vi "SW_Load_settings_to_main_tab.vi"(0 "Refnum in":T3=refnum, 1 "User Name":string="Admin", 7 "error in (no error)":errorcluster) -> (9 "VISA resource name":string, 12 "Vertical offset":dbl, 13 "Midfield segments outer radius, mm":i32=60, 14 "Cage diameter, mm":i32=180, 15 "Midfield segments starting angle":i32, 16 "Border segments starting angle":i32, 17 "Stimulus presets array":T2(array[cluster])=[{"Event type"=0, "Dur., s"=0.0, "Stim., s"=0.0, "Set/Clear"=FALSE, "TTL out N"=1, "Stim. has been set"=FALSE}, {"Event type"=0, "Dur., s"=0.0, "Stim., s"=0.0, "Set/Clear"=FALSE, "TTL out N"=1, "Stim. has been set"=FALSE}, {"Event type"=0, "Dur., s"=0.0, "Stim., s"=0.0, "Set/Clear"=FALSE, "TTL out N"=1, "Stim. has been set"=FALSE}, {"Event type"=0, "Dur., s"=0.0, "Stim., s"=0.0, "Set/Clear"=FALSE, "TTL out N"=1, "Stim. has been set"=FALSE}, {"Event type"=0, "Dur., s"=0.0, "Stim., s"=0.0, "Set/Clear"=FALSE, "TTL out N"=1, "Stim. has been set"=FALSE}, {"Event type"=0, "Dur., s"=0.0, "Stim., s"=0.0, "Set/Clear"=FALSE, "TTL out N"=1, "Stim. has been set"=FALSE}, {"Event type"=0, "Dur., s"=0.0, "Stim., s"=0.0, "Set/Clear"=FALSE, "TTL out N"=1, "Stim. has been set"=FALSE}, {"Event type"=0, "Dur., s"=0.0, "Stim., s"=0.0, "Set/Clear"=FALSE, "TTL out N"=1, "Stim. has been set"=FALSE}, {"Event type"=0, "Dur., s"=0.0, "Stim., s"=0.0, "Set/Clear"=FALSE, "TTL out N"=1, "Stim. has been set"=FALSE}, {"Event type"=0, "Dur., s"=0.0, "Stim., s"=0.0, "Set/Clear"=FALSE, "TTL out N"=1, "Stim. has been set"=FALSE}, {"Event type"=0, "Dur., s"=0.0, "Stim., s"=0.0, "Set/Clear"=FALSE, "TTL out N"=1, "Stim. has been set"=FALSE}, {"Event type"=0, "Dur., s"=0.0, "Stim., s"=0.0, "Set/Clear"=FALSE, "TTL out N"=1, "Stim. has been set"=FALSE}, {"Event type"=0, "Dur., s"=0.0, "Stim., s"=0.0, "Set/Clear"=FALSE, "TTL out N"=1, "Stim. has been set"=FALSE}, {"Event type"=0, "Dur., s"=0.0, "Stim., s"=0.0, "Set/Clear"=FALSE, "TTL out N"=1, "Stim. has been set"=FALSE}] {"Event type" items=["Stay for N seconds"]; "TTL out N" items=["1"=1, "2"=2, "1+2"=3]}, 19 "IO parameters cluster":T1, 20 "Refnum out":T3, 21 "Amount of midfield segments":i32=4, 23 "Mouse snout orientation swap?":bool, 24 "Amount of border segments":i32=8, 25 "Center segment outer radius, mm":i32=30, 27 "error out":errorcluster={"status"=TRUE, "code"=1, "source"="Dequeue Element in NI_LVConfig.lvlib:Read Value Without Comment.vi->NI_LVConfig.lvlib:Read Key (I32).vi->SW_Load_settings_to_main_tab.vi"})   [LabVIEW 2016]
uses:
  <vilib>/Utility/config.llb/Config Data RefNum.ctl
  <vilib>/Utility/config.llb/NI_LVConfig.lvlib
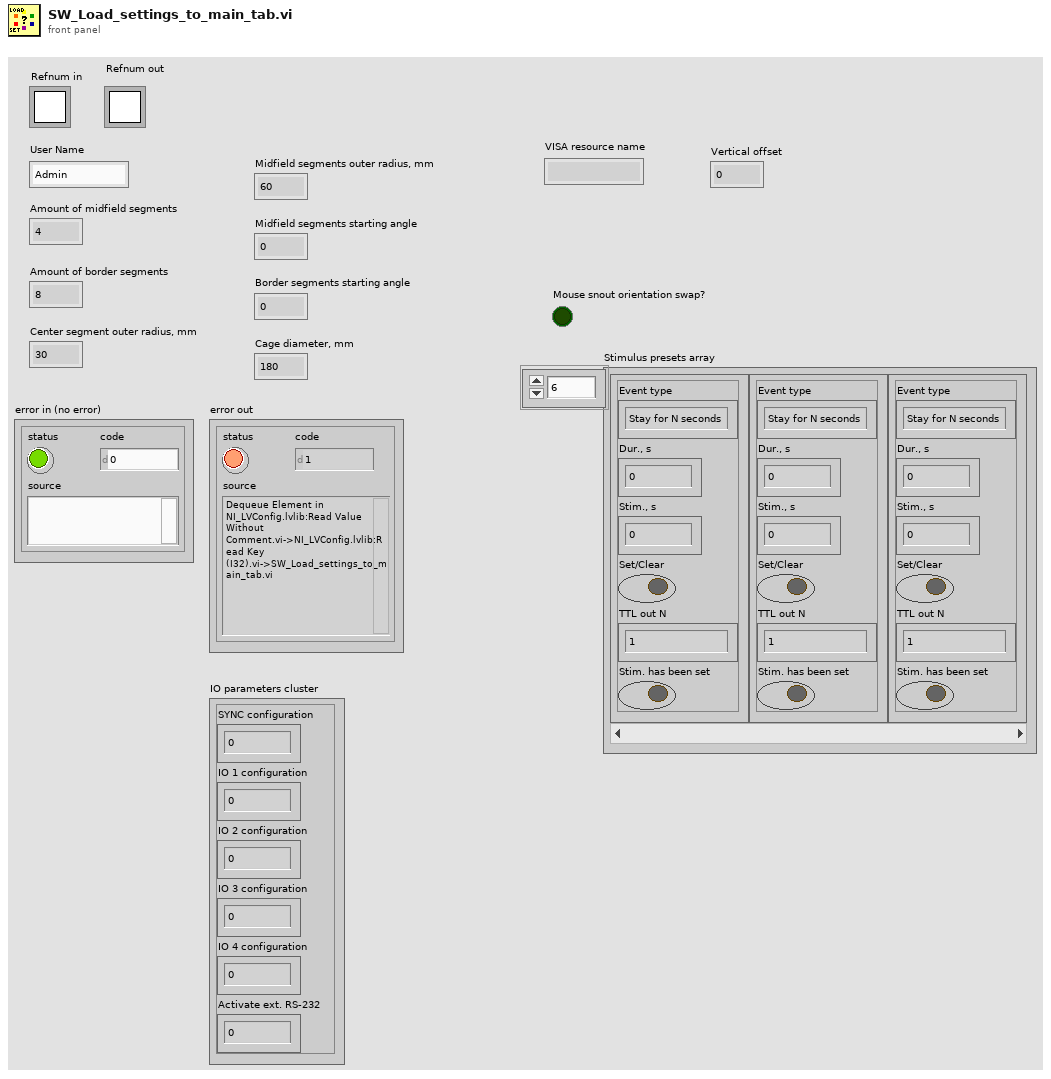
[diagram p1: front panel]
types:
  T1 = cluster{"SYNC configuration":u16, "IO 1 configuration":u16, "IO 2 configuration":u16, "IO 3 configuration":u16, "IO 4 configuration":u16, "Activate ext. RS-232":u16}
  T2 = cluster{"Event type":u16, "Dur., s":sgl, "Stim., s":sgl, "Set/Clear":bool, "TTL out N":u16, "Stim. has been set":bool}[]
  T3 = typedef "NI_LVConfig.lvlib/Config Data RefNum.ctl" = refnum<k1>
  T4 = cluster{"Event type":u16, "Time, s":sgl, "Stimulus, s":sgl, "Set/Clear":bool, "TTL out":u16, "Stim. has been set":bool}
  T5 = cluster{"array[0]":u16, "array[1]":u16, "array[2]":u16, "array[3]":u16, "array[4]":u16, "array[5]":u16, "array[6]":u16, "array[7]":u16, "array[8]":u16}
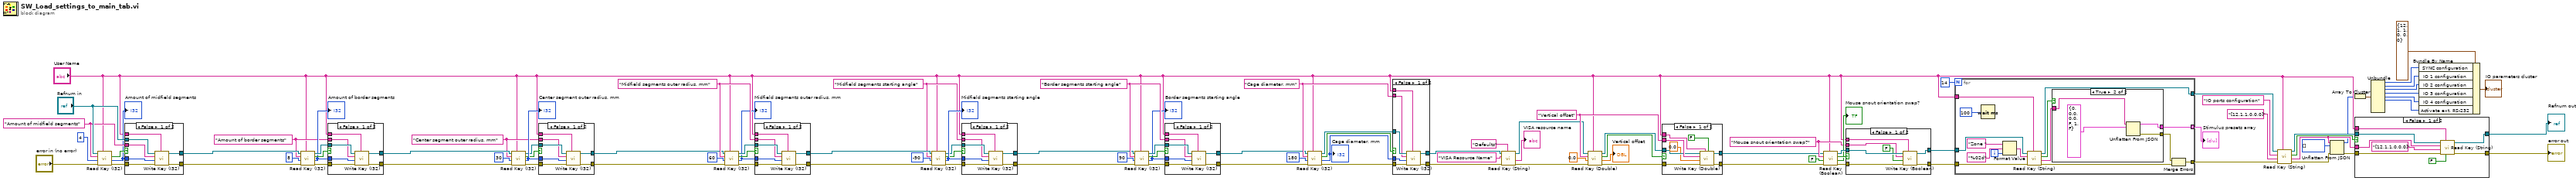
[diagram p0: block diagram]
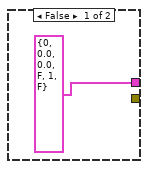
[diagram p4: hidden frame]
diagram:
  w26 = "Vertical offset" ("key")
  w39 = "Mouse snout orientation swap?"
  w51 = "Cage diameter, mm" ("key")
  w64 = "Border segments starting angle" ("key")
  w65 = "Midfield segments starting angle" ("key")
  w79 = "Midfield segments outer radius, mm" ("key")
  w82 = "Center segment outer radius, mm" ("key")
  w89 = "Amount of border segments" ("key")
  w100 = "Amount of midfield segments" ("key")
  n1 = call <vilib>:"Read Key (I32).vi"("section"="User Name", "error in (no error)"="error in (no error)", "default value"=4, "key"=w100, "refnum"="Refnum in") -> ("error out"=w98:errorcluster, "value"=w91:i32, "found?"=w102:bool)  [unwired: 3 in, 1 out]
  "Amount of midfield segments" <- w91
  n2 = case shown="False" w102 {
    tunnel: "User Name" -> [w109 _]
    tunnel: "Refnum in" -> [w110 w112]
    tunnel: w100 -> [w108 _]
    tunnel: w91 -> [w107 _]
    tunnel: w98 -> [w106 w111]
    tunnel: [w105 w111] -> w95
    tunnel: [w104 w112] -> w97
    frame False {
      n3 = call <vilib>:"Write Key (I32).vi"("section"=w109, "error in (no error)"=w106, "value"=w107, "key"=w108, "refnum"=w110) -> ("error out"=w105:errorcluster, "refnum out"=w104:T3)  [unwired: 4 in, 1 out]
    }
    frame True {
    }
  }
  n4 = call <vilib>:"Read Key (I32).vi"("section"="User Name", "error in (no error)"=w95, "default value"=8, "key"=w89, "refnum"=w97) -> ("error out"=w90:errorcluster, "value"=w92:i32, "found?"=w93:bool, "refnum out"=w94:T3)  [unwired: 3 in]
  "Amount of border segments" <- w92
  n5 = case shown="False" w93 {
    tunnel: "User Name" -> [w118 _]
    tunnel: w94 -> [w119 w121]
    tunnel: w89 -> [w117 _]
    tunnel: w92 -> [w116 _]
    tunnel: w90 -> [w115 w120]
    tunnel: [w114 w120] -> w84
    tunnel: [w113 w121] -> w83
    frame False {
      n6 = call <vilib>:"Write Key (I32).vi"("section"=w118, "error in (no error)"=w115, "value"=w116, "key"=w117, "refnum"=w119) -> ("error out"=w114:errorcluster, "refnum out"=w113:T3)  [unwired: 4 in, 1 out]
    }
    frame True {
    }
  }
  n7 = call <vilib>:"Read Key (I32).vi"("section"="User Name", "error in (no error)"=w84, "default value"=30, "key"=w82, "refnum"=w83) -> ("error out"=w88:errorcluster, "value"=w87:i32, "found?"=w86:bool, "refnum out"=w85:T3)  [unwired: 3 in]
  "Center segment outer radius, mm" <- w87
  n8 = case shown="False" w86 {
    tunnel: "User Name" -> [w127 _]
    tunnel: w85 -> [w128 w130]
    tunnel: w82 -> [w126 _]
    tunnel: w87 -> [w125 _]
    tunnel: w88 -> [w124 w129]
    tunnel: [w123 w129] -> w74
    tunnel: [w122 w130] -> w73
    frame False {
      n9 = call <vilib>:"Write Key (I32).vi"("section"=w127, "error in (no error)"=w124, "value"=w125, "key"=w126, "refnum"=w128) -> ("error out"=w123:errorcluster, "refnum out"=w122:T3)  [unwired: 4 in, 1 out]
    }
    frame True {
    }
  }
  n10 = call <vilib>:"Read Key (I32).vi"("section"="User Name", "error in (no error)"=w74, "default value"=60, "key"=w79, "refnum"=w73) -> ("error out"=w75:errorcluster, "value"=w76:i32, "found?"=w77:bool, "refnum out"=w78:T3)  [unwired: 3 in]
  "Midfield segments outer radius, mm" <- w76
  n11 = case shown="False" w77 {
    tunnel: "User Name" -> [w136 _]
    tunnel: w78 -> [w137 w139]
    tunnel: w79 -> [w135 _]
    tunnel: w76 -> [w134 _]
    tunnel: w75 -> [w133 w138]
    tunnel: [w132 w138] -> w67
    tunnel: [w131 w139] -> w66
    frame False {
      n12 = call <vilib>:"Write Key (I32).vi"("section"=w136, "error in (no error)"=w133, "value"=w134, "key"=w135, "refnum"=w137) -> ("error out"=w132:errorcluster, "refnum out"=w131:T3)  [unwired: 4 in, 1 out]
    }
    frame True {
    }
  }
  n13 = call <vilib>:"Read Key (I32).vi"("section"="User Name", "error in (no error)"=w67, "default value"=-90, "key"=w65, "refnum"=w66) -> ("error out"=w72:errorcluster, "value"=w71:i32, "found?"=w70:bool, "refnum out"=w69:T3)  [unwired: 3 in]
  "Midfield segments starting angle" <- w71
  n14 = case shown="False" w70 {
    tunnel: "User Name" -> [w145 _]
    tunnel: w69 -> [w146 w148]
    tunnel: w65 -> [w144 _]
    tunnel: w71 -> [w143 _]
    tunnel: w72 -> [w142 w147]
    tunnel: [w141 w147] -> w57
    tunnel: [w140 w148] -> w58
    frame False {
      n15 = call <vilib>:"Write Key (I32).vi"("section"=w145, "error in (no error)"=w142, "value"=w143, "key"=w144, "refnum"=w146) -> ("error out"=w141:errorcluster, "refnum out"=w140:T3)  [unwired: 4 in, 1 out]
    }
    frame True {
    }
  }
  n16 = call <vilib>:"Read Key (I32).vi"("section"="User Name", "error in (no error)"=w57, "default value"=90, "key"=w64, "refnum"=w58) -> ("error out"=w59:errorcluster, "value"=w60:i32, "found?"=w61:bool, "refnum out"=w62:T3)  [unwired: 3 in]
  "Border segments starting angle" <- w60
  n17 = case shown="False" w61 {
    tunnel: "User Name" -> [w154 _]
    tunnel: w62 -> [w155 w157]
    tunnel: w64 -> [w153 _]
    tunnel: w60 -> [w152 _]
    tunnel: w59 -> [w151 w156]
    tunnel: [w150 w156] -> w49
    tunnel: [w149 w157] -> w50
    frame False {
      n18 = call <vilib>:"Write Key (I32).vi"("section"=w154, "error in (no error)"=w151, "value"=w152, "key"=w153, "refnum"=w155) -> ("error out"=w150:errorcluster, "refnum out"=w149:T3)  [unwired: 4 in, 1 out]
    }
    frame True {
    }
  }
  n19 = call <vilib>:"Read Key (I32).vi"("section"="User Name", "error in (no error)"=w49, "default value"=180, "key"=w51, "refnum"=w50) -> ("error out"=w56:errorcluster, "value"=w55:i32, "found?"=w54:bool, "refnum out"=w53:T3)  [unwired: 3 in]
  "Cage diameter, mm" <- w55
  n20 = case shown="False" w54 {
    tunnel: "User Name" -> [w163 _]
    tunnel: w53 -> [w164 w166]
    tunnel: w51 -> [w162 _]
    tunnel: w55 -> [w161 _]
    tunnel: w56 -> [w160 w165]
    tunnel: [w159 w165] -> w48
    tunnel: [w158 w166] -> w46
    frame False {
      n21 = call <vilib>:"Write Key (I32).vi"("section"=w163, "error in (no error)"=w160, "value"=w161, "key"=w162, "refnum"=w164) -> ("error out"=w159:errorcluster, "refnum out"=w158:T3)  [unwired: 4 in, 1 out]
    }
    frame True {
    }
  }
  n22 = call <vilib>:"Read Key (String).vi"("section"="Defaults", "error in (no error)"=w48, "key"="VISA Resource Name", "refnum"=w46) -> ("error out"=w2:errorcluster, "value"=→"VISA resource name":string, "refnum out"=w1:T3)  [unwired: 4 in, 1 out]
  n23 = call <vilib>:"Read Key (Double).vi"("section"="User Name", "error in (no error)"=w2, "default value"=0.0, "key"=w26, "refnum"=w1) -> ("error out"=w31:errorcluster, "value"=→"Vertical offset":dbl, "found?"=w29:bool, "refnum out"=w27:T3)  [unwired: 3 in]
  n24 = case shown="False" w29 {
    tunnel: [w172 w175] -> w32
    tunnel: [w173 w176] -> w33
    tunnel: w31 -> [w174 w176]
    tunnel: "User Name" -> [w171 _]
    tunnel: w26 -> [w170 _]
    tunnel: w27 -> [w168 w175]
    frame False {
      n25 = call <vilib>:"Write Key (Double).vi"("use system decimal point (T)"=FALSE ("value"), "section"=w171, "error in (no error)"=w174, "value"=0.0, "key"=w170, "refnum"=w168) -> ("error out"=w173:errorcluster, "refnum out"=w172:T3)  [unwired: 3 in, 1 out]
    }
    frame True {
    }
  }
  n26 = call <vilib>:"Read Key (Boolean).vi"("section"="User Name", "error in (no error)"=w33, "default value"=FALSE, "key"=w39, "refnum"=w32) -> ("error out"=w42:errorcluster, "value"=→"Mouse snout orientation swap?":bool, "found?"=w41:bool, "refnum out"=w43:T3)  [unwired: 3 in]
  n27 = case shown="False" w41 {
    tunnel: w43 -> [w181 w185]
    tunnel: [w180 w185] -> w36
    tunnel: [w182 w184] -> w35
    tunnel: w42 -> [w183 w184]
    tunnel: "User Name" -> [w179 _]
    tunnel: w39 -> [w178 _]
    frame False {
      n28 = call <vilib>:"Write Key (Boolean).vi"("section"=w179, "error in (no error)"=w183, "value"=FALSE, "key"=w178, "refnum"=w181) -> ("error out"=w182:errorcluster, "refnum out"=w180:T3)  [unwired: 4 in, 1 out]
    }
    frame True {
    }
  }
  n29 = for {
    N: 14 -> [_]
    tunnel: w36 -> [w198]
    tunnel: [w197] -> w25
    tunnel: "User Name" -> [w196]
    tunnel: w35 -> [w194]
    tunnel: [w188] -> w24
    tunnel: [w191] -> w34 mode=indexing
    i -> [w189]
    n30 = Wait (ms)(milliseconds to wait=u32 100) -> ()  [unwired: 1 out]
    n31 = Format Value(string ("")="Zone ", format string="%02d", value (0)=w189) -> (output string=w195:string)
    n32 = call <vilib>:"Read Key (String).vi"("section"=w196, "error in (no error)"=w194, "key"=w195, "refnum"=w198) -> ("error out"=w193:errorcluster, "value"=w192:string, "found?"=w190:bool, "refnum out"=w197:T3)  [unwired: 4 in]
    n33 = case shown="True" w190 {
      tunnel: w192 -> [_ w205]
      tunnel: [T4 {"Event type"=0, "Time, s"=0.0, "Stimulus, s"=0.0, "Set/Clear"=FALSE, "TTL out"=1, "Stim. has been set"=FALSE} ("Cluster of the stimuls settings") w204] -> w191
      tunnel: [_ w203] -> w187
      frame False {
      }
      frame True {
        n34 = Unflatten From JSON(JSON string=w205, type and defaults=T4 {"Event type"=0, "Time, s"=0.0, "Stimulus, s"=0.0, "Set/Clear"=FALSE, "TTL out"=1, "Stim. has been set"=FALSE} ("Cluster of the stimuls settings")) -> (value=w204:T4, error out=w203:errorcluster)  [unwired: 5 in]
      }
    }
    n35 = Merge Errors(w187, w193) -> (w188:errorcluster)
  }
  "Stimulus presets array" <- w34
  n36 = call <vilib>:"Read Key (String).vi"("section"="User Name", "error in (no error)"=w24, "default value"="[12,1,1,0,0,0]" ("IO parameters string"), "key"="IO ports configuration", "refnum"=w25) -> ("error out"=w15:errorcluster, "value"=w16:string, "found?"=w19:bool, "refnum out"=w18:T3)  [unwired: 3 in]
  n37 = Unflatten From JSON(JSON string=w16, type and defaults=u16[] [] ("array"), error in (no error)=w15) -> (value=w13:u16[], error out=w14:errorcluster)  [unwired: 4 in]
  n38 = Array To Cluster(array=w13) -> (cluster=w11:T5)
  n39 = case shown="False" w19 {
    tunnel: w18 -> [w211 w215]
    tunnel: [w210 w215] -> w22
    tunnel: [w212 w214] -> w23
    tunnel: w14 -> [w213 w214]
    tunnel: "User Name" -> [w209 _]
    tunnel: w16 -> [w208 _]
    frame False {
      n40 = call <vilib>:"Read Key (String).vi"("read raw string? (F)"=FALSE ("value"), "section"=w209, "error in (no error)"=w213, "default value"="[12,1,1,0,0,0]" ("IO parameters string"), "key"=w208, "refnum"=w211) -> ("error out"=w212:errorcluster, "refnum out"=w210:T3)  [unwired: 2 in, 2 out]
    }
    frame True {
    }
  }
  "error out" <- w23
  "Refnum out" <- w22
  n41 = Unbundle(w11) -> ("array[0]"=w10:u16, "array[1]"=w9:u16, "array[2]"=w8:u16, "array[3]"=w7:u16, "array[4]"=w6:u16, "array[5]"=w5:u16)  [unwired: 3 out]
  n42 = Bundle By Name(cluster=T1 {"SYNC configuration"=12, "IO 1 configuration"=1, "IO 2 configuration"=1, "IO 3 configuration"=0, "IO 4 configuration"=0, "Activate ext. RS-232"=0} ("Sync parameters cluster output"), "SYNC configuration"=w10, "IO 1 configuration"=w9, "IO 2 configuration"=w8, "IO 3 configuration"=w7, "IO 4 configuration"=w6, "Activate ext. RS-232"=w5) -> (→"IO parameters cluster":T1)
